vi "PH_Sequencer.PC StateTiming.vi"(0 "i ref in":refnum<vi>, 3 "State":T1 items=["no info", "off/false/out", "on/true/in", "Failure", "Alarm", "Status 1", "Status 2", "Status 3"], 4 "not linked?":bool, 5 "error in (no error)":errorcluster) -> (14 "i ref out":refnum<vi>, 19 "error out":errorcluster)   [LabVIEW 2014, in "PH_Sequencer.lvlib"]
doc: "This VI writes the state of the timing instance to own attributes and the GUI elements."
uses:
  PH_Sequencer.lvlib
  PH_Basics/PH_StatusHandler/PH_StatusHandler.Status.ctl
  PH_Basics/PH_StatusHandler/PH_StatusHandler.lvlib
  PH_Basics/PH_Common/PH_Common.lvlib
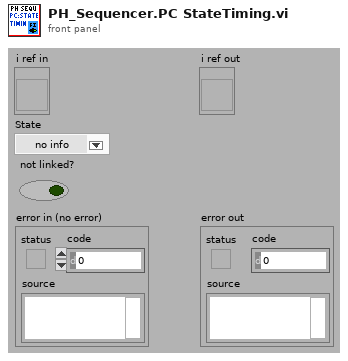
[diagram p1: front panel]
types:
  T1 = typedef "PH_StatusHandler.lvlib/PH_StatusHandler.Status.ctl" = i16
  T2 = typedef "PH_Sequencer.lvlib/PH_Sequencer.i attribute.ctl" = cluster{"GUI Refs":cluster{"Main Off":refnum<vi>, "Fire":refnum<vi>, "Status":refnum<vi>, "Ready":refnum<vi>, "Waiting Time":refnum<vi>, "Timeout":refnum<vi>, "PPMA Ready":refnum<vi>, "Sequencer SM State":refnum<vi>, "PPPA Ready":refnum<vi>, "Calorimeter":refnum<vi>, "Beamline Ready":refnum<vi>, "Clear Beamline":refnum<vi>, "Linkage PPMA Rods":refnum<vi>, "Linkage Current PA":refnum<vi>, "Linkage Current MA":refnum<vi>, "Timing Ready":refnum<vi>, "State Timing":refnum<vi>, "Force Timing":refnum<vi>, "PSDB Shot Comment":refnum<vi>, "State PA Backreflection":refnum<vi>, "Beamline Z6 Ready":refnum<vi>, "Clear Z6 Beamline":refnum<vi>, "Sequence length":refnum<vi>, "Timing Mode":refnum<vi>, "Slow Trigger Settings":refnum<vi>, "Experiment Description":refnum<vi>, "State PSDB":refnum<vi>, "PSDB Ready":refnum<vi>, "Set PSDB Settings":refnum<vi>, "Get PSDB Info":refnum<vi>, "Take Snapshot":refnum<vi>, "Shottype":refnum<vi>, "Experiment":refnum<vi>, "Phase Frontends":refnum<vi>, "PP 45mm PILC in use":refnum<vi>}, "Status Info":cluster{"Machine Status":T1, "WaitingTime":i32, "Timeout":bool}, "Readyness":cluster{"Ready to shot":bool, "PPMA Ready":bool, "PPPA Ready":bool, "BL Ready":bool, "Timing Ready":bool, "BL Z6 Ready":bool, "PSDBReady":bool}, "Instancenames":cluster{"PPMA Rods":string, "PP Current Meas":string, "PH Beamline Chief":string, "PA Backrefl Meas":string, "Z6 Beamline Chief":string}, "Data to read":bool, "Calorimeter":cluster{"Instancename":string, "On":bool, "linked":bool}, "Linkage":cluster{"PPMA Rods":bool, "PP Current Meas":bool, "PHELIX Beamline Chief":bool, "PA Backrefl Meas":bool, "Z6 Beamline Chief":bool}, "Timing":cluster{"Instance":string, "linked":bool, "Status":T1, "Timing Mode":T3, "Slow Trigger Settings":T4, "Info available":cluster{"ext SlowTrigger":bool, "T2":bool, "Mode":bool, "Delay Slow Trigger":bool, "Phase FEs":bool}, "FE Phase":T5}, "Service ID R2S":i32, "PSDB":cluster{"Controller Instance":string, "Controller Status":T1, "Controller linked":bool, "Settings acknowledged":bool, "Current Experiment ID":i16, "Current Shot Type":i16, "Current Comment":string, "Remember Settings":bool, "Write 2 early":bool}, "PSDB Data":cluster{"Main Off?":bool, "Sequence Length":dbl, "Sequence startet":timestamp}, "6P 4Q Positions":cluster{"Instancename":string, "linked":bool, "Position":T6}[], "PUs":T7[]}
  T3 = typedef "PH_Timing.lvlib/PH_Timing.Timing Mode.ctl" = cluster{"T2":i16, "Modeselector":enum32{"10 Hz", "0.5 Hz", "Shot"}}
  T4 = typedef "PH_Timing.lvlib/PH_Timing.Slow Trigger Settings.ctl" = cluster{"Delay":dbl, "externally triggered?":bool}
  T5 = typedef "PH_Timing.lvlib/PH_Timing.Phase FEs.ctl" = cluster{"Phase":dbl}
  T6 = typedef "PH_4_Pos_Selector.lvlib/PH_4_Pos_Selector.Position Selector.ctl" = u16
  T7 = typedef "PH_Sequencer.lvlib/PH_Sequencer.Head.ctl" = cluster{"PowerUnit":T8, "GUI Ref":refnum<vi>, "Information":T9, "linked?":bool, "GUI Ref Current Voltage":refnum<vi>}
  T8 = typedef "PH_PP_Common.lvlib/PH_PP_Common.PUs.ctl" = enum16{"no Info", "PA-19mm-1", "PA-19mm-2", "PA-45mm-PILC", "PA-45mm-MAIN", "MA-PU-1", "MA-PU-2", "MA-PU-3", "MA-PU-4", "MA-PU-5", "MA-PU-6", "MA-FR", "MA-PILC", "PA-45mm-DP"}
  T9 = typedef "PH_Sequencer.lvlib/PH_Sequencer.PU Information.ctl" = cluster{"State":T1, "Waiting Time [s]":dbl, "PU State SM":T10, "PU Timeout SM":T10}
  T10 = typedef "PH_PowerUnit_BaseClass.lvlib/PH_PowerUnit_BaseClass.SM States.ctl" = enum16{".", "Stand by", "Switch PU on", "Configure", "Set Default Voltage", "Set STANDBY", "Set READY", "Wait for Shot Cmd", "Open Dump Rods", "Open Ross Relais", "Close Ross Relais", "Switch PSU on", "Switch PSU off", "Charge", "Switch GD Channel on", "Close Dump Rods", "Rods-TO", "RR-TO", "PSU-TO", "Trigger-TO"}
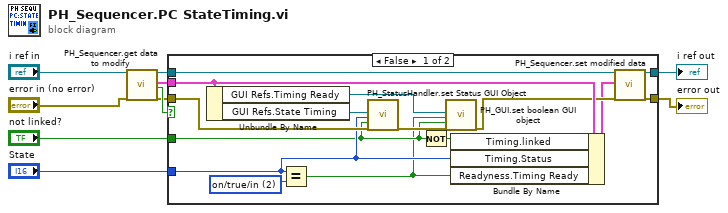
[diagram p0: block diagram]
diagram:
  n1 = call "PH_Sequencer.get data to modify.vi"("i ref in"="i ref in", "error in (no error)"="error in (no error)") -> ("i ref out"=w4:refnum<vi>, "i attribute"=w8:T2, "timed out"=w10:bool, "error out"=w6:errorcluster)  [unwired: 14 in]
  n2 = case shown="False" w10 {
    tunnel: w4 -> [w25 w27]
    tunnel: [w24 w27] -> w5
    tunnel: w6 -> [w20 w26]
    tunnel: [w23 w26] -> w7
    tunnel: w8 -> [w19 _]
    tunnel: "State" -> [w17 _]
    tunnel: "not linked?" -> [w14 _]
    frame False {
      w22 = T1 2 items=["no info", "off/false/out", "on/true/in", "Failure", "Alarm", "Status 1", "Status 2", "Status 3"] ("y")
      n3 = Unbundle By Name(w19) -> ("GUI Refs.Timing Ready"=w15:refnum<vi>, "GUI Refs.State Timing"=w18:refnum<vi>)
      n4 = Equal?(x=w17, y=w22) -> (x = y?=w13:bool)
      n5 = call "PH_StatusHandler.set Status GUI Object.vi"("PH Status Ref"=w18, "Value"=w17, "Blinking (false)"=w14, "error in (no error)"=w20) -> ("error out"=w16:errorcluster)  [unwired: 15 in]
      n6 = Not(x=w14) -> (.not. x?=w21:bool)
      n7 = call "PH_GUI.set boolean GUI object.vi"("Boolean Knob GUI Ref"=w15, "Value"=w13, "Blinking? (false)"=w14, "error in (no error)"=w16) -> ("error out"=w12:errorcluster)  [unwired: 15 in]
      n8 = Bundle By Name(cluster=w19, "Timing.linked"=w21, "Timing.Status"=w17, "Readyness.Timing Ready"=w13) -> (w11:T2)
      n9 = call "PH_Sequencer.set modified data.vi"("i ref in"=w25, "i attribute"=w11, "error in (no error)"=w12) -> ("i ref out"=w24:refnum<vi>, "error out"=w23:errorcluster)  [unwired: 15 in]
    }
    frame True {
    }
  }
  "error out" <- w7
  "i ref out" <- w5
